vi "AutoLin Grafik aufbereiten FT-IR.vi"(10 "Sollwerte":sgl[](array[numeric]), 11 "Istwerte":sgl[](array[numeric])) -> (3 "XY-Graph (roh/lin)":cluster{"eine Kurve":sgl[], dbl[]}[](array[cluster]))   [LabVIEW 2020, in "Linearisierung v2.lvlib"]
doc: "Bereitet die Kalibrierdaten in ein Array aus Einzelkurven (Cluster aus X-Array, Y-Array) für die Darstellung in einem XY-Graphen für folgende Kurven auf:\n\nabs. Fehler (ppm) der Rohwerte des Messgerätes\nabs. Fehler (ppm) der linearisierten Messwerte\nNull-Linie, entspricht Sollwerten\n\nLin-Eingangsdaten: 2D-Array (SGL) mit Konzentrationswerten in ppm\n 1. Spalte: Gasteiler\n 2. Spalte Messgerät\n\nLin-Polynom: enthält unter anderem die Polynokoeffizienten (Typdefinition, Cluster)"
uses:
  Linearisierung v2.lvlib
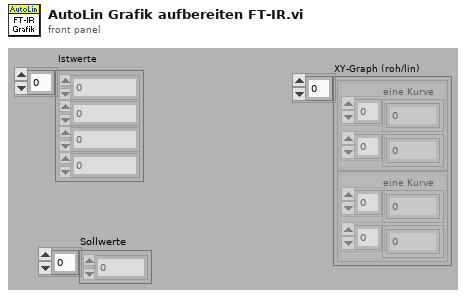
[diagram p1: front panel]
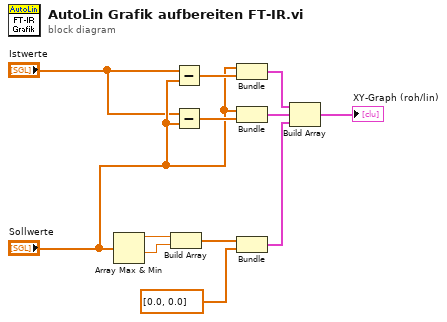
[diagram p0: block diagram]
diagram:
  n1 = Array Max & Min(array="Sollwerte") -> (max value=w6:sgl, min value=w5:sgl)  [unwired: 2 out]
  n2 = Build Array(w6, w5) -> (w4:sgl[])
  n3 = Subtract(x="Istwerte", y="Sollwerte") -> (x-y=w11:sgl[])
  n4 = Subtract(x="Istwerte", y="Sollwerte") -> (x-y=w12:sgl[])
  n5 = Bundle("Sollwerte"="Sollwerte", w11) -> (w8:cluster{"Sollwerte":sgl[], sgl[]})  [unwired: 1 in]
  n6 = Bundle("Sollwerte"="Sollwerte", w12) -> (w9:cluster{"Sollwerte":sgl[], sgl[]})  [unwired: 1 in]
  n7 = Bundle(w4, sgl[] [0.0, 0.0]) -> (w3:cluster{sgl[], sgl[]})  [unwired: 1 in]
  n8 = Build Array(w8, w9, w3) -> (→"XY-Graph (roh/lin)":cluster{"Sollwerte":sgl[], sgl[]}[])
